vi "csm_setpoint_and_ramp_lumikki.vi"() -> ()   [LabVIEW 2009]
uses:
  <vilib>/Analysis/7linalg.llb/Real Kronecker Product.vi
  <vilib>/Utility/file.llb/Write To Spreadsheet File (DBL).vi
  <vilib>/Analysis/NI_AALPro.lvlib
panel:
  out "Waveform Graph 2":dbl[][](graph)
  in  "Interval/Buffer Parameters":T1={"Sample interval - ms (2)"=2.0, "Buffer Length (1000)"=1000, "No. of Buffers (0)"=0} {"Sample interval - ms (2)" min=0.2 format="%.1f"}
  in  "folder":string
  in  "Measurement ID":string
  out "ramp start armed":bool
  out "logging":bool
  out "Block 5 active":bool
  in  "Go to block 6":bool
  in  "Go to block 5":bool
  in  "Enter the experiment \nsetup values:":T2 {"Set Point" format="%.2f"; "Ramp Amplitude" format="%.2f"; "Ramp Rate" format="%.2f"; "Set Point Time" format="%.2f"}
  out "Current ramp amplitude":dbl[](array[numeric]) format="%.2f"
  out "Current ramp rate":dbl[](array[numeric]) format="%.2f"
  in  "Choose channel to apply\nthe ramp:":u16[](array[ring]) items=["Channel 1", "Channel 2", "Channel 3", "Channel 4"]
  out "Block 4 active":bool
  in  "Go to block 4":bool
  out "Block 3 active":bool
  in  "Enter setpoint\nvalues:":T2 {"Set Point" format="%.2f"; "Ramp Amplitude" format="%.2f"; "Ramp Rate" format="%.2f"; "Set Point Time" format="%.2f"}
  in  "Choose channel to apply\nthe setpoint":u16[](array[ring]) items=["Channel 1", "Channel 2", "Channel 3", "Channel 4"]
  out "Current setpoint\n machine":dbl[](array[numeric]) format="%.2f"
  out "Duration to reach \nthe setpoint":dbl[](array[numeric]) format="%.2f"
  in  "Machine found:":i32[](listbox)
  out "Block 2 active":bool
  out "Block 1 active":bool
  in  "stop":bool
  in  "Go to block 2":bool
  in  "Go to block 3":bool
  # "1: Initialization"
  # "4: Set Ramp parameters"
  # "2: Set Setpoint parameters"
  # "ch1 position\nch2 load\nch3 digital position\nch4 external"
  # "this stages sets the crosshead\n to an initial position or force \nvalue in a given time"
  # "Save data to target:"
  # "ch1 position\nch2 load\nch3 digital position\nch4 external"
  # "START THE EXPERIMENT ->"
  # "MOVE TO SETPOINT ->"
  # "3: Moving to setpoint"
  # "5: Stop exp and log"
  # "STOP THE EXPERIMENT ->"
  # "datalogger internal \npreferences:"
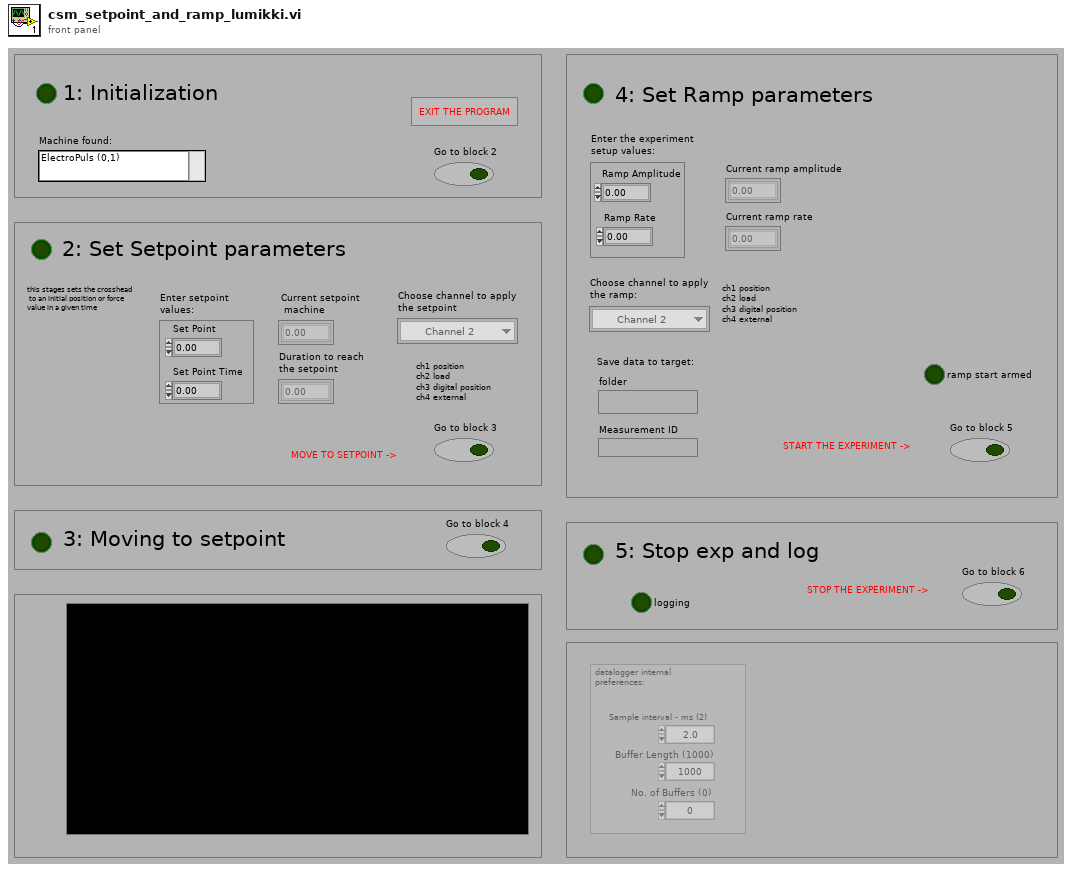
[diagram p1: front panel]
types:
  T1 = cluster{"Sample interval - ms (2)":dbl, "Buffer Length (1000)":i32, "No. of Buffers (0)":i32}
  T2 = cluster{"Set Point":dbl, "Set Point Time":dbl, "Ramp Amplitude":dbl, "Ramp Rate":dbl}
  T3 = cluster{"Name":string, "Type":i32, "SI Full Scale":dbl, "Full Scale":dbl, "Units String":string, "Display Format":string, "Gauge Length":dbl}[][]
  T4 = cluster{"Device ID":i32, "Device Name":string, "Device Type":i32}[]
  T5 = typedef "NI_Matrix.lvlib/RealMatrix.ctl" = dbl[][]
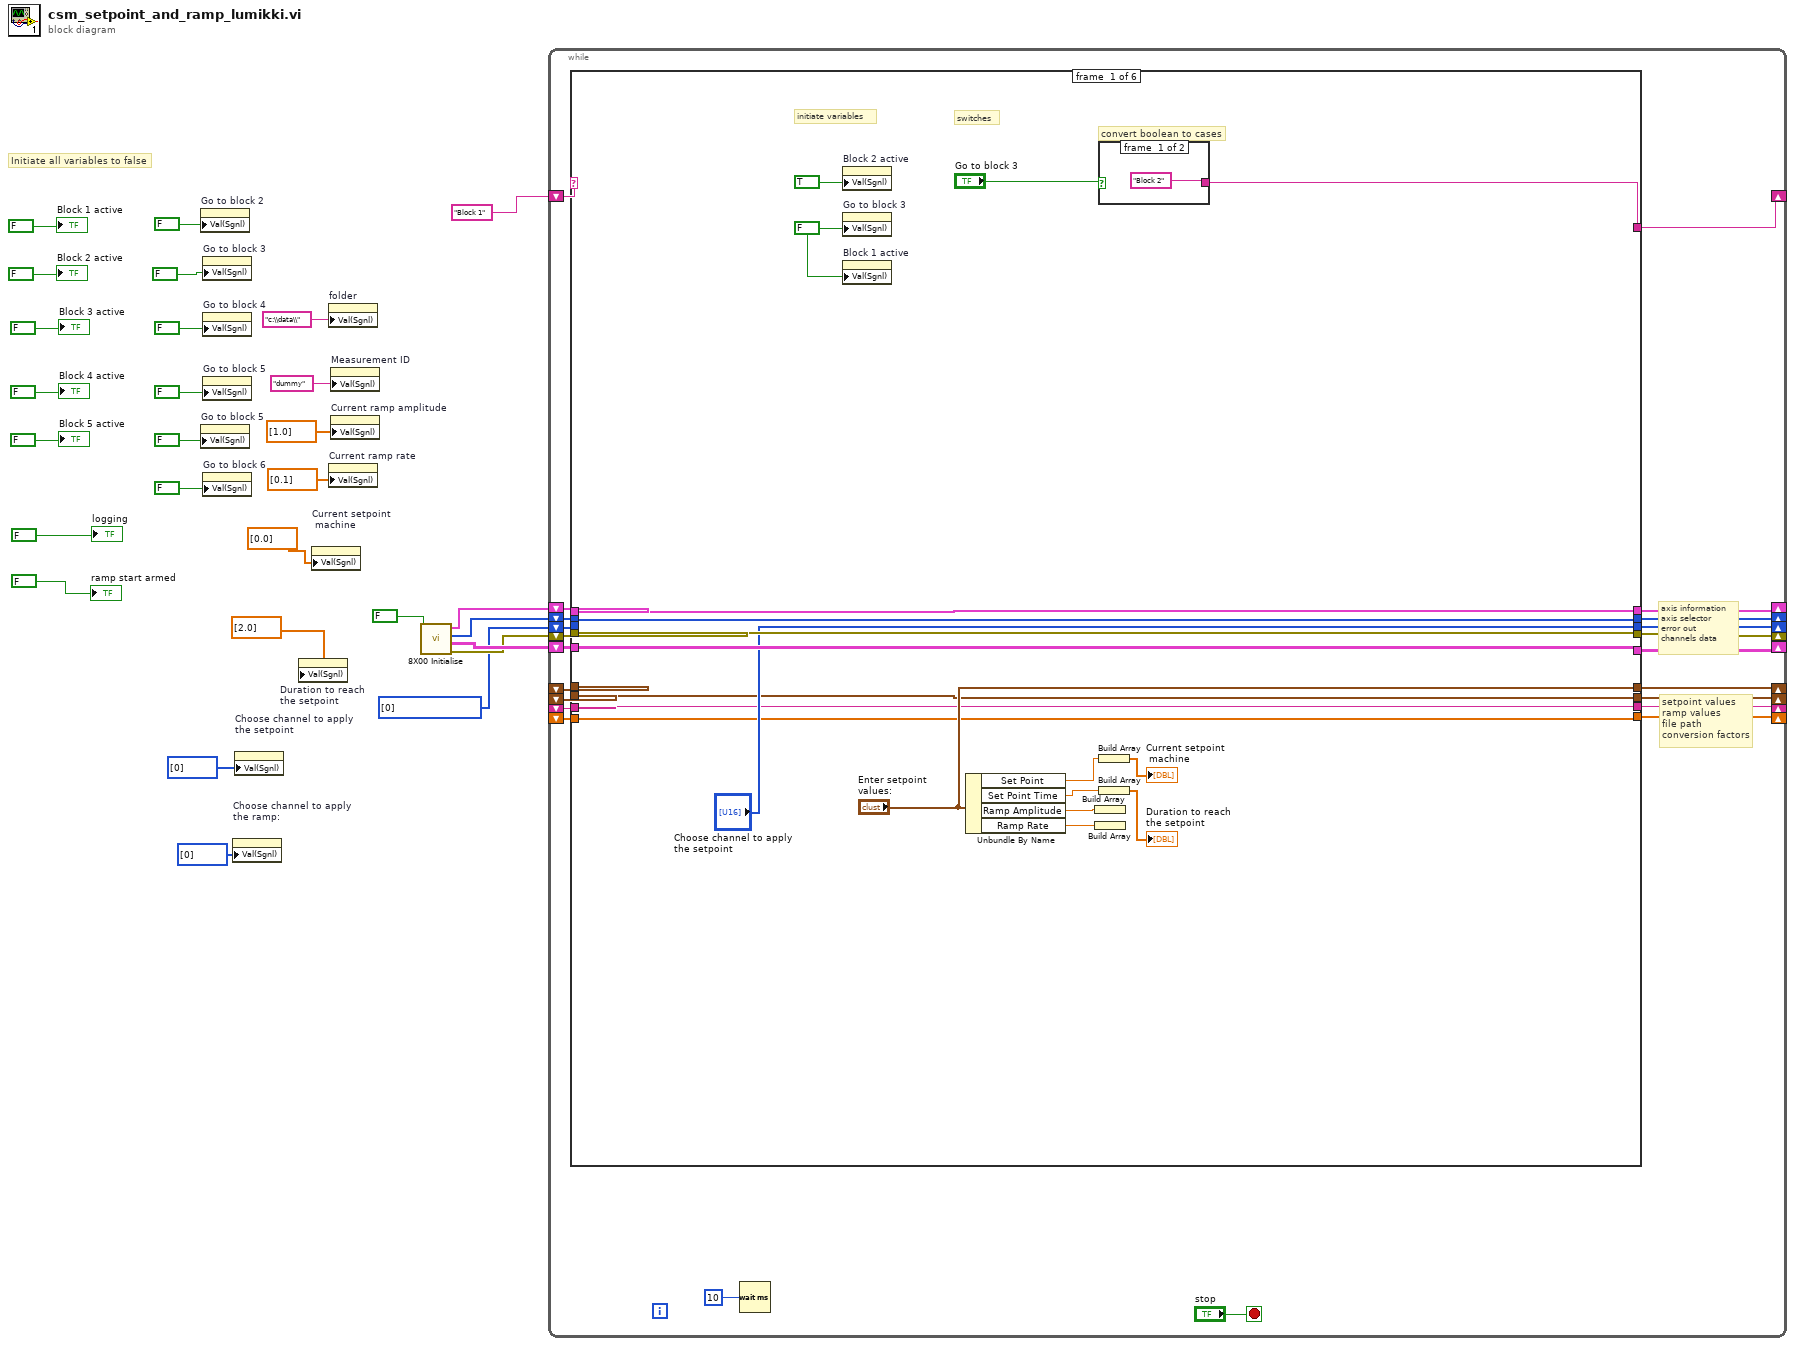
[diagram p0: block diagram]
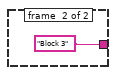
[diagram p2: hidden frame]
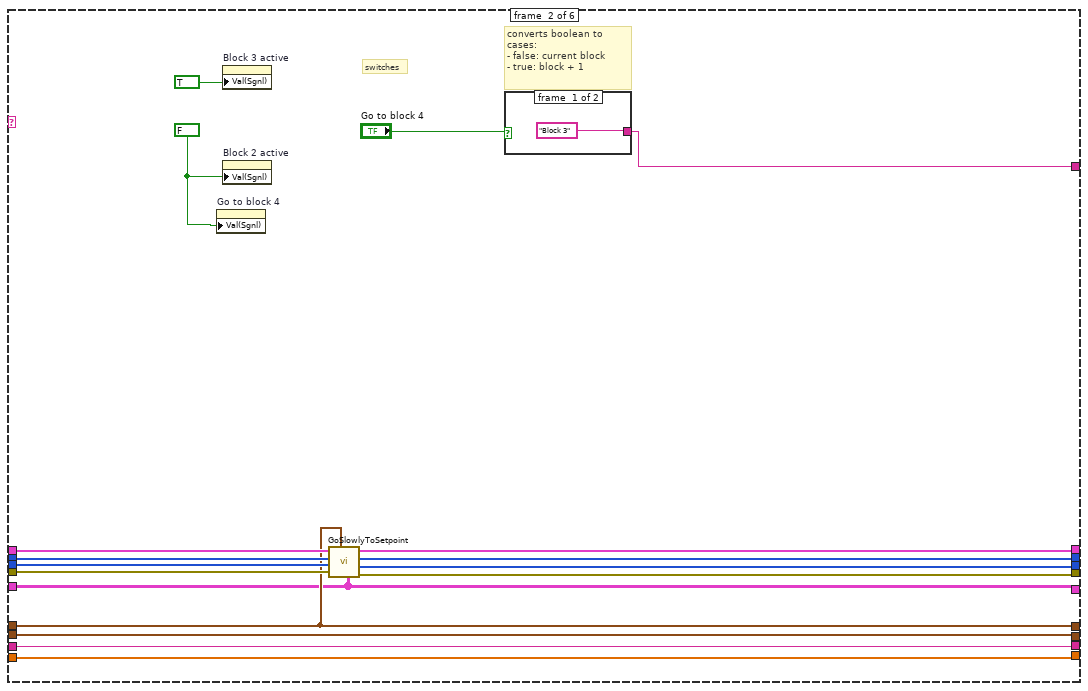
[diagram p3: hidden frame]
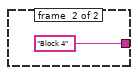
[diagram p4: hidden frame]
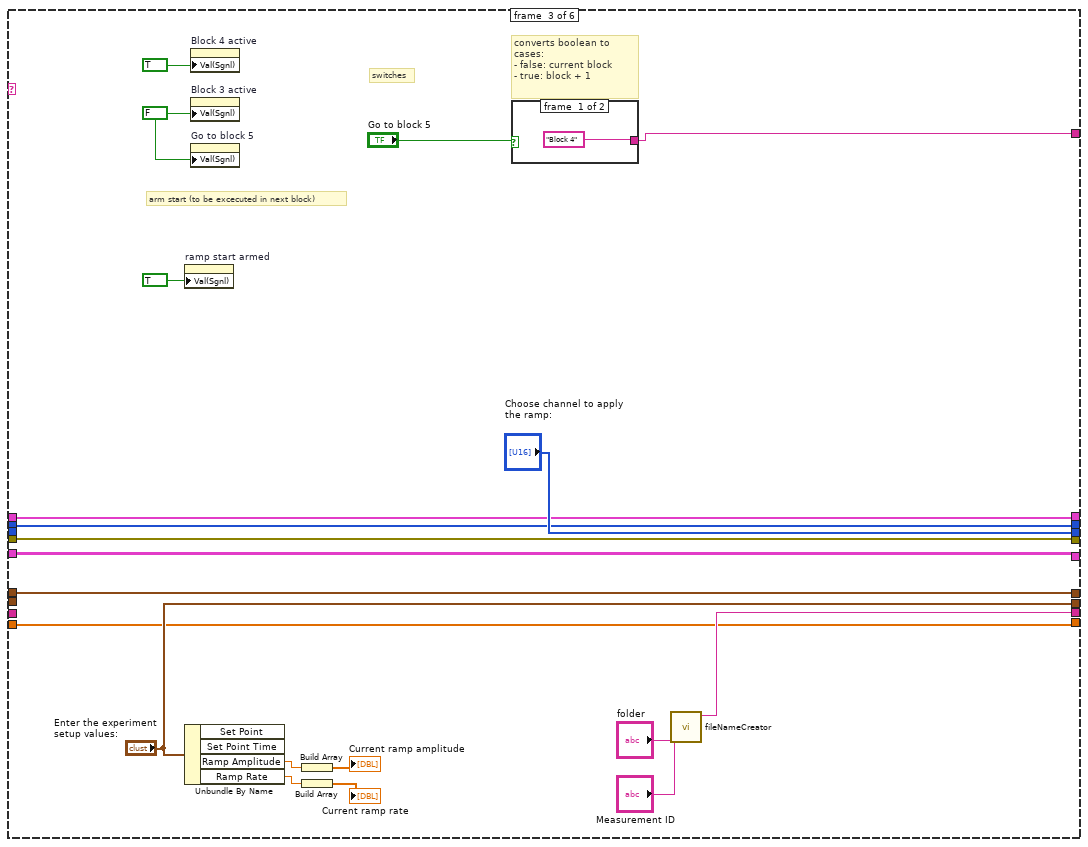
[diagram p5: hidden frame]
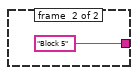
[diagram p6: hidden frame]
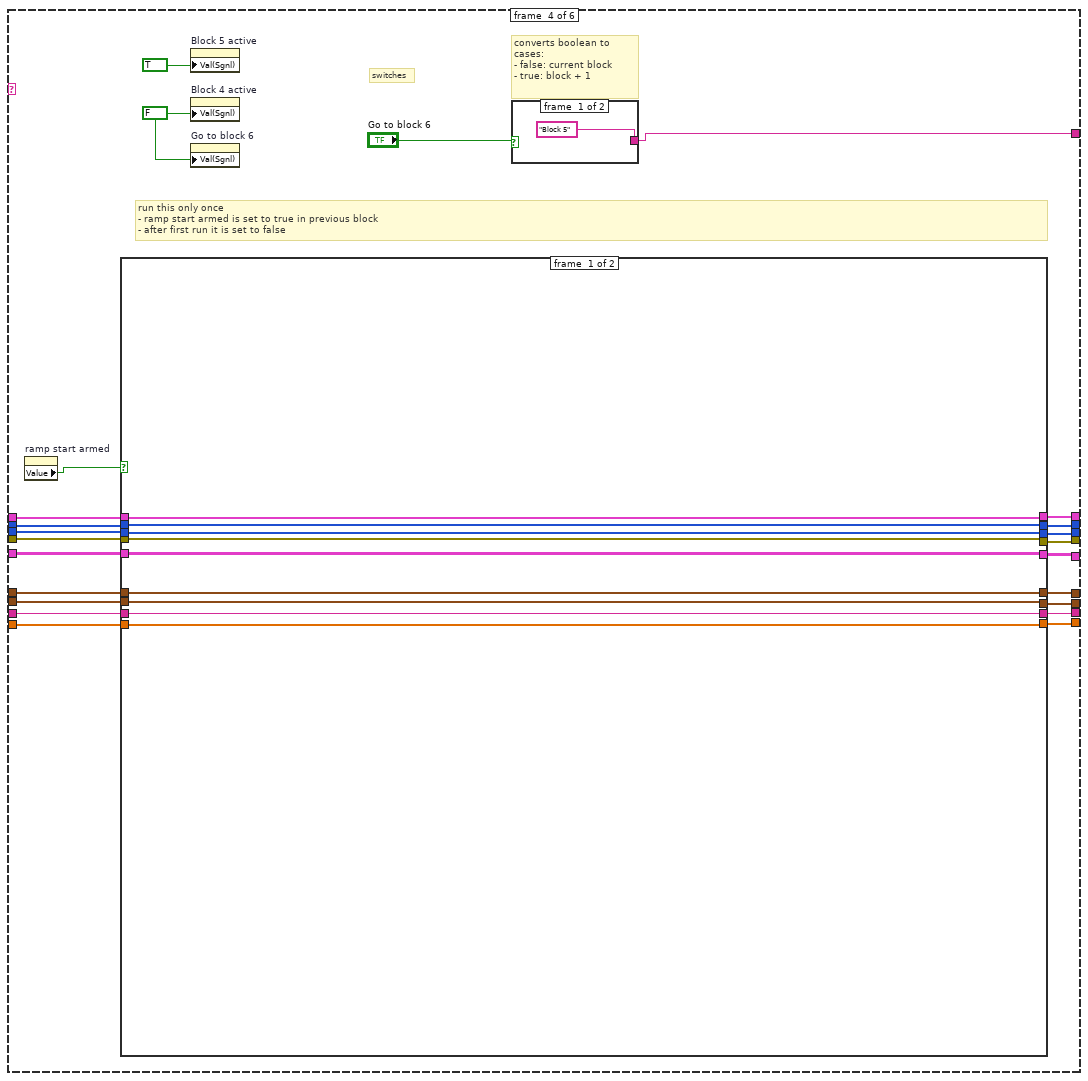
[diagram p7: hidden frame]
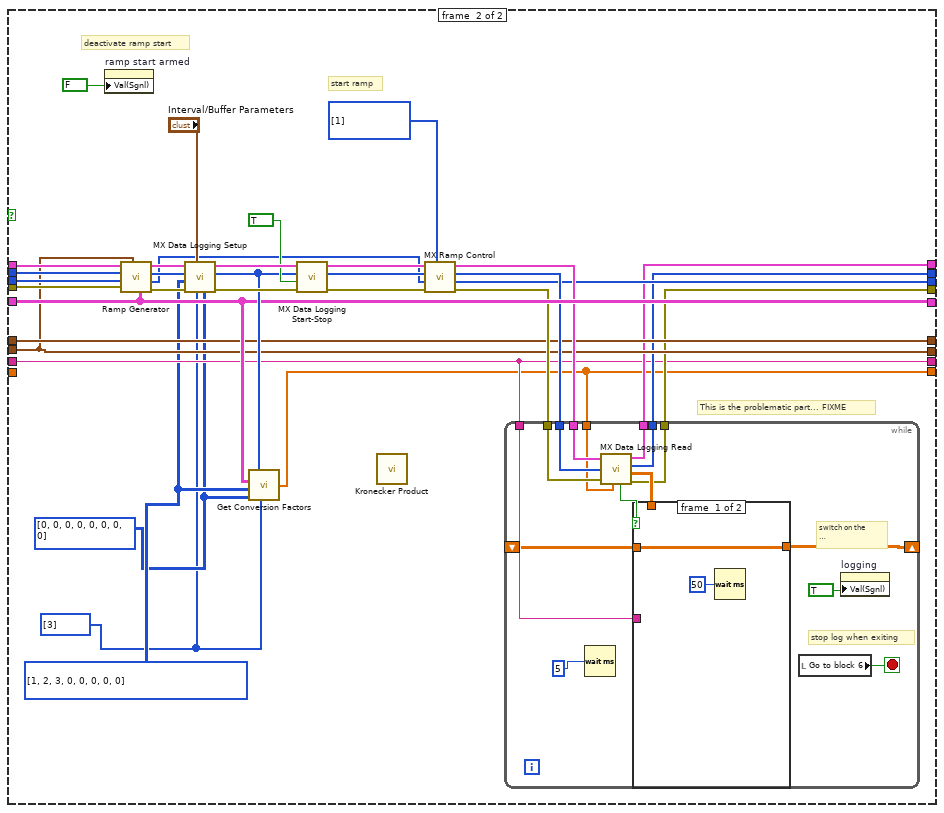
[diagram p8: hidden frame]
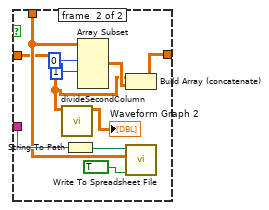
[diagram p9: hidden frame]
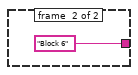
[diagram p10: hidden frame]
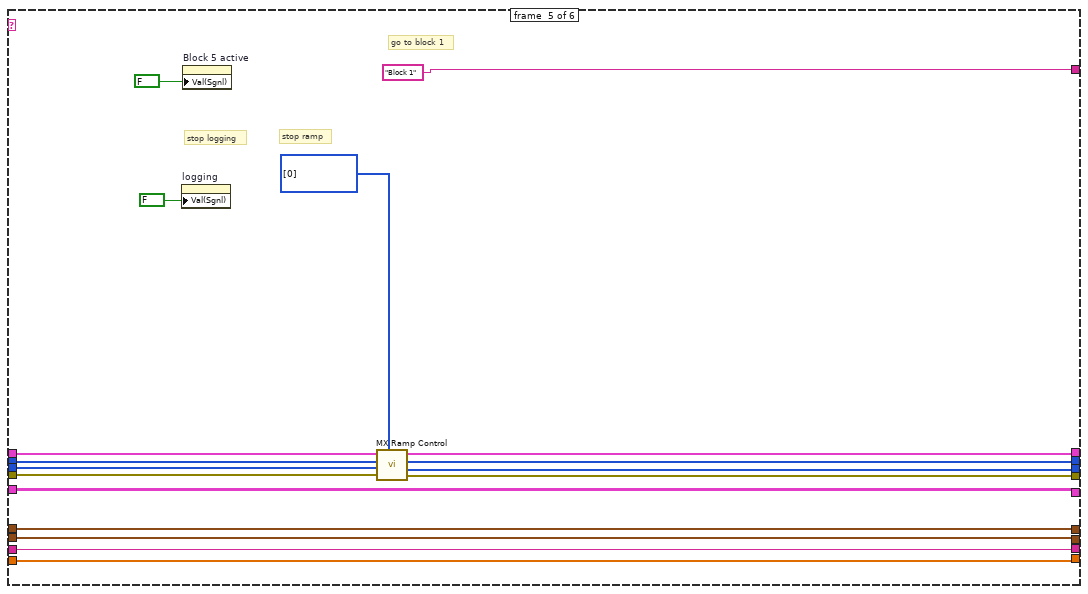
[diagram p11: hidden frame]
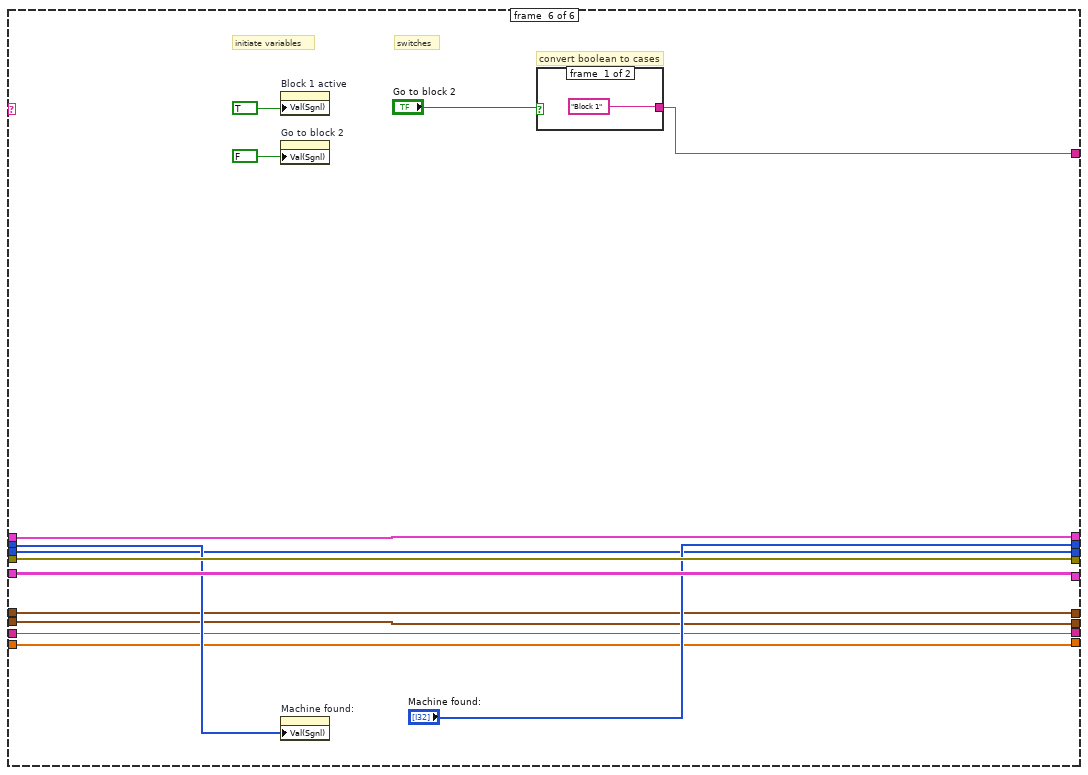
[diagram p12: hidden frame]
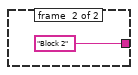
[diagram p13: hidden frame]
diagram:
  w18 = u16[] [0] items=["Channel 1", "Channel 2", "Channel 3", "Channel 4"] ("Choose channel to apply\nthe setpoint")
  # "Initiate all variables to false"
  n1 = property on="Go to block 2" class="Bool (strict)"("Val(Sgnl)"=FALSE ("Value (Signaling)")) -> ()  [unwired: 2 in, 2 out]
  n2 = property on="Go to block 5" class="Bool (strict)"("Val(Sgnl)"=FALSE ("Value (Signaling)")) -> ()  [unwired: 2 in, 2 out]
  n3 = property on="Go to block 3" class="Bool (strict)"("Val(Sgnl)"=FALSE ("Value (Signaling)")) -> ()  [unwired: 2 in, 2 out]
  n4 = property on="Go to block 4" class="Bool (strict)"("Val(Sgnl)"=FALSE ("Value (Signaling)")) -> ()  [unwired: 2 in, 2 out]
  n5 = property on="Go to block 5" class="Bool (strict)"("Val(Sgnl)"=FALSE ("Value (Signaling)")) -> ()  [unwired: 2 in, 2 out]
  n6 = property on="Go to block 6" class="Bool (strict)"("Val(Sgnl)"=FALSE ("Value (Signaling)")) -> ()  [unwired: 2 in, 2 out]
  n7 = property on="Choose channel to apply\nthe ramp:" class="Arr (strict)"("Val(Sgnl)"=u16[] [0] ("Value (Signaling)")) -> ()  [unwired: 2 in, 2 out]
  n8 = property on="Choose channel to apply\nthe setpoint" class="Arr (strict)"("Val(Sgnl)"=u16[] [0] ("Value (Signaling)")) -> ()  [unwired: 2 in, 2 out]
  n9 = property on="Duration to reach \nthe setpoint" class="Arr (strict)"("Val(Sgnl)"=dbl[] [2.0] ("Value (Signaling)")) -> ()  [unwired: 2 in, 2 out]
  n10 = property on="Current setpoint\n machine" class="Arr (strict)"("Val(Sgnl)"=dbl[] [0.0] ("Value (Signaling)")) -> ()  [unwired: 2 in, 2 out]
  n11 = property on="folder" class="Str"("Val(Sgnl)"="c:\\data\\" ("Value (Signaling)")) -> ()  [unwired: 2 in, 2 out]
  n12 = property on="Current ramp rate" class="Arr (strict)"("Val(Sgnl)"=dbl[] [0.1] ("Value (Signaling)")) -> ()  [unwired: 2 in, 2 out]
  n13 = property on="Measurement ID" class="Str"("Val(Sgnl)"="dummy" ("Value (Signaling)")) -> ()  [unwired: 2 in, 2 out]
  n14 = property on="Current ramp amplitude" class="Arr (strict)"("Val(Sgnl)"=dbl[] [1.0] ("Value (Signaling)")) -> ()  [unwired: 2 in, 2 out]
  n15 = call "8X00 Initialise.vi"("Reset?"=FALSE) -> ("error out"=w19:errorcluster, "Channel Data"=w20:T3, "Axis Selector"=w21:i32[], "Axis Information"=w22:T4)  [unwired: 3 in]
  n16 = while {
    shift-right: [w47] -> _
    shift-left: "Block 1" -> [w48]
    shift-right: [w42] -> _
    shift-left: w22 -> [w46]
    shift-right: [w41] -> _
    shift-left: w21 -> [w45]
    shift-right: [w39] -> _
    shift-left: w20 -> [w44]
    shift-right: [w40] -> _
    shift-left: w19 -> [w43]
    shift-right: [w37] -> _
    shift-left: w18 -> [w38]
    shift-right: [w36] -> _
    shift-left: _ -> [w35]
    shift-right: [w34] -> _
    shift-left: _ -> [w33]
    shift-right: [w32] -> _
    shift-left: _ -> [w31]
    shift-right: [w30] -> _
    shift-left: _ -> [w29]
    stop <- "stop" stop-if-true
    # "setpoint values\nramp values\nfile path\nconversion factors"
    # "axis information\naxis selector\nerror out\nchannels data"
    n17 = case shown="\"Block 4\"" w48 {
      tunnel: [w68 w75 w103 w132 "Block 1" w237] -> w47
      tunnel: w46 -> [w65 w85 w91 w127 w218 w234]
      tunnel: w45 -> [w64 w84 w92 w126 w217 w230]
      tunnel: w44 -> [w63 w76 w94 w131 w210 w233]
      tunnel: w43 -> [w62 w82 w93 w125 w215 w232]
      tunnel: [w65 w81 w91 w122 w214 w234] -> w42
      tunnel: [w64 w80 w92 w113 w213 "Machine found:"] -> w41
      tunnel: [w62 w78 w93 w120 w211 w232] -> w40
      tunnel: [w63 w76 w94 w129 w210 w233] -> w39
      tunnel: w38 -> [_ w83 _ w124 w216 w228]
      tunnel: ["Choose channel to apply\nthe setpoint" w79 "Choose channel to apply\nthe ramp:" w121 w212 w228] -> w37
      tunnel: ["Enter setpoint\nvalues:" w77 w102 w115 w222 w227] -> w36
      tunnel: w35 -> [_ w77 w102 w116 w222 w227]
      tunnel: [w52 w73 w96 w118 w220 w225] -> w34
      tunnel: w33 -> [w52 w73 _ w119 w220 w225]
      tunnel: [w53 w74 "Enter the experiment \nsetup values:" w114 w221 w226] -> w32
      tunnel: w31 -> [w53 w74 _ w117 w221 w226]
      tunnel: [w51 w72 w95 w123 w208 w224] -> w30
      tunnel: w29 -> [w51 w72 w95 w128 w208 w224]
      frame #0 {
        w66 = FALSE ("Value (Signaling)")
        # "convert boolean to cases"
        # "switches"
        # "initiate variables"
        n18 = property on="Block 2 active" class="Bool (strict)"("Val(Sgnl)"=TRUE ("Value (Signaling)")) -> ()  [unwired: 2 in, 2 out]
        n19 = property on="Go to block 3" class="Bool (strict)"("Val(Sgnl)"=w66) -> ()  [unwired: 2 in, 2 out]
        n20 = property on="Block 1 active" class="Bool (strict)"("Val(Sgnl)"=w66) -> ()  [unwired: 2 in, 2 out]
        n21 = Unbundle By Name("Enter setpoint\nvalues:") -> ("Set Point"=w59:dbl, "Set Point Time"=w58:dbl, "Ramp Amplitude"=w60:dbl, "Ramp Rate"=w57:dbl)
        n22 = Build Array(w60) -> ()  [unwired: 1 out]
        n23 = Build Array(w57) -> ()  [unwired: 1 out]
        n24 = case shown="True" "Go to block 3" {
          tunnel: ["Block 2" "Block 3"] -> w68
          frame #0 {
          }
          frame #1 {
          }
        }
        n25 = Build Array(w59) -> (→"Current setpoint\n machine":dbl[])
        n26 = Build Array(w58) -> (→"Duration to reach \nthe setpoint":dbl[])
      }
      frame #1 {
        w86 = FALSE ("Value (Signaling)")
        # "converts boolean to cases:\n- false: current block\n- true: block + 1"
        # "switches"
        n27 = property on="Go to block 4" class="Bool (strict)"("Val(Sgnl)"=w86) -> ()  [unwired: 2 in, 2 out]
        n28 = property on="Block 3 active" class="Bool (strict)"("Val(Sgnl)"=TRUE ("Block 1 active")) -> ()  [unwired: 2 in, 2 out]
        n29 = property on="Block 2 active" class="Bool (strict)"("Val(Sgnl)"=w86) -> ()  [unwired: 2 in, 2 out]
        n30 = call "GoSlowlyToSetpoint.vi"("Channel Data"=w76, "Input cluster"=w77, "error in (no error)"=w82, "Channels"=w83, "Axis Selector"=w84, "Axis Information"=w85) -> ("Error Out"=w78:errorcluster, "Channels Out"=w79:u16[], "Axis Selector Out"=w80:i32[], "Axis Information Out"=w81:T4)  [unwired: 2 in]
        n31 = case shown="False" "Go to block 4" {
          tunnel: ["Block 3" "Block 4"] -> w75
          frame #0 {
          }
          frame #1 {
          }
        }
      }
      frame #2 {
        w109 = FALSE ("Value (Signaling)")
        # "arm start (to be excecuted in next block)"
        # "converts boolean to cases:\n- false: current block\n- true: block + 1"
        # "switches"
        n32 = property on="ramp start armed" class="Bool (strict)"("Val(Sgnl)"=TRUE ("Value (Signaling)")) -> ()  [unwired: 2 in, 2 out]
        n33 = Unbundle By Name("Enter the experiment \nsetup values:") -> ("Ramp Amplitude"=w108:dbl, "Ramp Rate"=w106:dbl)  [unwired: 2 out]
        n34 = property on="Block 4 active" class="Bool (strict)"("Val(Sgnl)"=TRUE ("Block 1 active")) -> ()  [unwired: 2 in, 2 out]
        n35 = property on="Block 3 active" class="Bool (strict)"("Val(Sgnl)"=w109) -> ()  [unwired: 2 in, 2 out]
        n36 = property on="Go to block 5" class="Bool (strict)"("Val(Sgnl)"=w109) -> ()  [unwired: 2 in, 2 out]
        n37 = Build Array(w108) -> (→"Current ramp amplitude":dbl[])
        n38 = Build Array(w106) -> (→"Current ramp rate":dbl[])
        n39 = case shown="False" "Go to block 5" {
          tunnel: ["Block 4" "Block 5"] -> w103
          frame #0 {
          }
          frame #1 {
          }
        }
        n40 = call "fileNameCreator.vi"("folder"="folder", "Measurement ID"="Measurement ID") -> ("concatenated string"=w96:string)  [unwired: 9 in]
      }
      frame #3 {
        w134 = FALSE ("Value (Signaling)")
        # "run this only once \n- ramp start armed is set to true in previous block\n- after first run it is set to false"
        # "converts boolean to cases:\n- false: current block\n- true: block + 1"
        # "switches"
        n41 = property on="ramp start armed" class="Bool (strict)"() -> ("Value"=w130:bool)  [unwired: 2 in, 2 out]
        n42 = case shown="True" w130 {
          tunnel: w125 -> [w142 w177]
          tunnel: w131 -> [w141 w164]
          tunnel: w127 -> [w144 w176]
          tunnel: w126 -> [w136 w175]
          tunnel: w124 -> [w143 w165]
          tunnel: [w141 w164] -> w129
          tunnel: [w142 w150] -> w120
          tunnel: [w143 w156] -> w121
          tunnel: [w144 w152] -> w122
          tunnel: [w140 w148] -> w123
          tunnel: w128 -> [w140 _]
          tunnel: w119 -> [w137 w149]
          tunnel: [w137 w149] -> w118
          tunnel: w117 -> [w138 w153]
          tunnel: w116 -> [w139 w154]
          tunnel: [w139 w154] -> w115
          tunnel: [w138 w153] -> w114
          tunnel: [w136 w151] -> w113
          frame #0 {
          }
          frame #1 {
            w145 = i32[] [3] ("Number of Columns")
            w146 = i32[][] [[0, 0, 0, 0, 0, 0, 0, 0]] items=["Feedback", "Direct Auxilary"] ("Column Types")
            w147 = i32[][] [[1, 2, 3, 0, 0, 0, 0, 0]] items=["Not Used", "Channel 1/Logging time", "Channel 2/Controlling command", "Channel 3/Controlling error", "Channel 4/Elapsed quarter-cycle counter", "Total accumulated quarter-cycle counter", "Elapsed segment counter", "Total accumulated segment counter", "Servovalve drive", "Block count", "Uncompensated servovalve drive", "Geometric compensation output 1", "Geometric compensation output 2", "Re-Sampling Filter 1", "Re-Sampling Filter 2", "Re-Sampling Filter 3", "Re-Sampling Filter 4", "Outer cascaded controller output", "Delta_P or acceleration compensation (Raw)", "Auxiliary input from the front of the IAC", "Waveform identifier", "Reserved", "Digital I/O and sample playback actions", "Reserved", "Motor current (EIB only)", "Motor instantaneous power (EIB only)", "Motot filtered power (EIB only)", "Motor speed (EIB only)", "Motor viscous loss (EIB only)"] ("Column Channels")
            w155 = u16[] [1] items=["Stop", "Start or continue", "Hold", "Continue", "Return ramp to set level at fixed rate", "Reserved", "Reserved", "Start Random without demand hold", "Start Random with demand hold", "Prepare Random Start without demand hold", "Prepare Random Start with demand hold", "Unslave", "Reserved", "Reserved", "Start Sample Data Playback or Resume", "Prepare for Start of Sample Data", "Reserved", "Reserved", "Resume Playback", "Start an electromechanical frame return"] ("Ramp Control")
            # "This is the problematic part... FIXME"
            # "deactivate ramp start"
            # "start ramp"
            n43 = property on="ramp start armed" class="Bool (strict)"("Val(Sgnl)"=FALSE ("Value (Signaling)")) -> ()  [unwired: 2 in, 2 out]
            n44 = call "Ramp Generator.vi"("Channel Data"=w164, "Input cluster"=w153, "error in (no error)"=w177, "Channels"=w165, "Axis Selector"=w175, "Axis Information"=w176) -> ("Error Out"=w170:errorcluster, "Channels Out"=w157:u16[], "Axis Selector Out"=w171:i32[], "Axis Information Out"=w172:T4)  [unwired: 2 in]
            n45 = call "MX Data Logging Setup.vi"("Column Types"=w146, "Number of Columns"=w145, "Interval/Buffer Parameters"="Interval/Buffer Parameters", "error in (no error)"=w170, "Column Channels"=w147, "Axis Selector"=w171, "Axis Information"=w172) -> ("error out"=w168:errorcluster, "Axis Selector copy"=w166:i32[], "Axis Information out"=w169:T4)  [unwired: 1 out]
            n46 = call "Get Conversion Factors.vi"("Axis Selector"=w166, "Channel Data"=w164, "Column Channels"=w147, "Column Types"=w146, "Number of Columns"=w145) -> ("Conversion Factors"=w148:dbl[])
            n47 = call "MX Data Logging Start-Stop.vi"("error in (no error)"=w168, "Start (T)"=TRUE, "Axis Selector"=w166, "Axis Information"=w169) -> ("error out"=w161:errorcluster, "Axis Selector copy"=w162:i32[], "Axis Information out"=w163:T4)  [unwired: 4 in]
            n48 = call-poly <vilib>:"Kronecker Product.vi"() -> ()  [unwired: 10 in, 2 out]
            n49 = call "MX Ramp Control.vi"("Ramp Control"=w155, "error in (no error)"=w161, "Channels In"=w157, "Axis Selector In"=w162, "Axis Information In"=w163) -> ("error out"=w160:errorcluster, "Channels Out"=w156:u16[], "Axis Selector Out"=w159:i32[], "Axis Information Out"=w158:T4)  [unwired: 2 in]
            n50 = while {
              tunnel: [w183] -> w150
              tunnel: [w184] -> w151
              tunnel: w160 -> [w187]
              tunnel: w148 -> [w186]
              tunnel: w159 -> [w188]
              tunnel: w158 -> [w189]
              tunnel: [w182] -> w152
              tunnel: w149 -> [w181]
              shift-right: [w179] -> _
              shift-left: _ -> [w178]
              stop <- w191 stop-if-true
              # "stop log when exiting"
              # "switch on the \n\nlogging light"
              n51 = Wait (ms)(milliseconds to wait=u32 5) -> ()  [unwired: 1 out]
              n52 = call "MX Data Logging Read.vi"("Axis Information"=w189, "Axis Selector"=w188, "error in (no error)"=w187, "Conversion Values (100)"=w186) -> ("Axis Information copy"=w182:T4, "Axis Selector copy"=w184:i32[], "Data Available"=w185:bool, "Collected Data - Eng Units"=w190:dbl[][], "error out"=w183:errorcluster)  [unwired: 2 out]
              n53 = case shown="True" w185 {
                tunnel: w190 -> [_ w201]
                tunnel: w181 -> [_ w202]
                tunnel: [w193 w197] -> w179
                tunnel: w178 -> [w193 w196]
                frame #0 {
                  n54 = Wait (ms)(milliseconds to wait=u32 50) -> ()  [unwired: 1 out]
                }
                frame #1 {
                  n55 = call "divideSecondColumn.vi"("Real Matrix"=w196) -> ("submatrix"=→"Waveform Graph 2":T5)  [unwired: 10 in]
                  n56 = String To Path(string=w202) -> (path=w204:path)
                  n57 = Array Subset(array=w201, index (row)=0 ("index"), length (row)=1 ("length")) -> (w198:dbl[][])  [unwired: 2 in]
                  n58 = Build Array (concatenate)(w196, w198) -> (w197:dbl[][])
                  n59 = call-poly <vilib>:"Write To Spreadsheet File.vi"("append to file? (new file:F)"=TRUE, "2D data"=w201, "file path (dialog if empty)"=w204) -> ()  [unwired: 5 in, 1 out]
                }
              }
              n60 = local read "Go to block 6"() -> (w191:bool)
              n61 = property on="logging" class="Bool (strict)"("Val(Sgnl)"=TRUE ("Value (Signaling)")) -> ()  [unwired: 2 in, 2 out]
            }
          }
        }
        n62 = property on="Block 5 active" class="Bool (strict)"("Val(Sgnl)"=TRUE ("Block 1 active")) -> ()  [unwired: 2 in, 2 out]
        n63 = property on="Block 4 active" class="Bool (strict)"("Val(Sgnl)"=w134) -> ()  [unwired: 2 in, 2 out]
        n64 = property on="Go to block 6" class="Bool (strict)"("Val(Sgnl)"=w134) -> ()  [unwired: 2 in, 2 out]
        n65 = case shown="False" "Go to block 6" {
          tunnel: ["Block 5" "Block 6"] -> w132
          frame #0 {
          }
          frame #1 {
          }
        }
      }
      frame #4 {
        w219 = u16[] [0] items=["Stop", "Start or continue", "Hold", "Continue", "Return ramp to set level at fixed rate", "Reserved", "Reserved", "Start Random without demand hold", "Start Random with demand hold", "Prepare Random Start without demand hold", "Prepare Random Start with demand hold", "Unslave", "Reserved", "Reserved", "Start Sample Data Playback or Resume", "Prepare for Start of Sample Data", "Reserved", "Reserved", "Resume Playback", "Start an electromechanical frame return"] ("Ramp Control")
        # "go to block 1"
        # "stop ramp"
        # "stop logging"
        n66 = property on="logging" class="Bool (strict)"("Val(Sgnl)"=FALSE ("Value (Signaling)")) -> ()  [unwired: 2 in, 2 out]
        n67 = property on="Block 5 active" class="Bool (strict)"("Val(Sgnl)"=FALSE ("Value (Signaling)")) -> ()  [unwired: 2 in, 2 out]
        n68 = call "MX Ramp Control.vi"("Ramp Control"=w219, "error in (no error)"=w215, "Channels In"=w216, "Axis Selector In"=w217, "Axis Information In"=w218) -> ("error out"=w211:errorcluster, "Channels Out"=w212:u16[], "Axis Selector Out"=w213:i32[], "Axis Information Out"=w214:T4)  [unwired: 2 in]
      }
      frame #5 {
        # "convert boolean to cases"
        # "switches"
        # "initiate variables"
        n69 = property on="Block 1 active" class="Bool (strict)"("Val(Sgnl)"=TRUE ("Block 1 active")) -> ()  [unwired: 2 in, 2 out]
        n70 = property on="Go to block 2" class="Bool (strict)"("Val(Sgnl)"=FALSE ("Value (Signaling)")) -> ()  [unwired: 2 in, 2 out]
        n71 = property on="Machine found:" class="LstBox (strict)"("Val(Sgnl)"=w230) -> ()  [unwired: 2 in, 2 out]
        n72 = case shown="True" "Go to block 2" {
          tunnel: ["Block 1" "Block 2"] -> w237
          frame #0 {
          }
          frame #1 {
          }
        }
      }
    }
    n73 = Wait (ms)(milliseconds to wait=u32 10) -> ()  [unwired: 1 out]
  }
  "Block 1 active" <- FALSE ("Block 1 active")
  "Block 2 active" <- FALSE ("Block 2 active")
  "Block 3 active" <- FALSE ("Block 2 active")
  "Block 4 active" <- FALSE ("Block 4 active")
  "Block 5 active" <- FALSE ("Block 4 active")
  "logging" <- FALSE ("Block 4 active")
  "ramp start armed" <- FALSE ("activate start")
